vi "Get_FIFO.vi"(8 "error in (no error)":errorcluster) -> (0 "error out":errorcluster, 2 "TrajectoryFIFO":T1)   [LabVIEW 2019]
uses:
  <vilib>/Utility/error.llb/Error Cluster From Error Code.vi
  <vilib>/ErrorRing/Error Ring.xnode
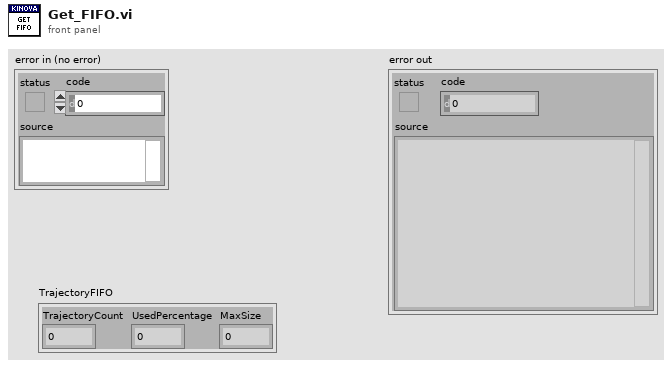
[diagram p1: front panel]
types:
  T1 = cluster{"TrajectoryCount":u32, "UsedPercentage":sgl, "MaxSize":u32}
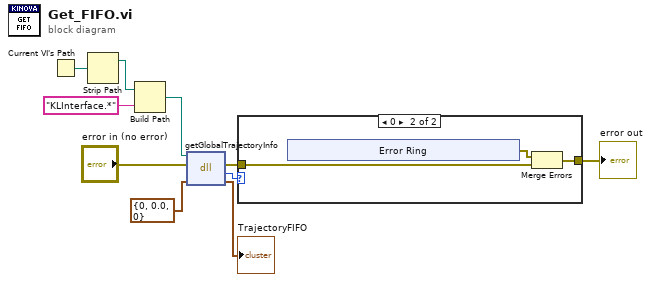
[diagram p0: block diagram]
diagram:
  n1 = Current VI's Path() -> (path=w7:path)
  n2 = Strip Path(path=w7) -> (stripped path=w6:path)  [unwired: 1 out]
  n3 = Build Path(base path=w6, name or relative path="KLInterface.*") -> (appended path=w2:path)
  n4 = dll-call lib="C:/Users/mcjssdcc/Documents/Kinova-Labview-Interface/KLInterface.dll" fn="getGlobalTrajectoryInfo"(path in=w2, error in="error in (no error)", "point"=T1 {"TrajectoryCount"=0, "UsedPercentage"=0.0, "MaxSize"=0} ("TrajectoryFIFO")) -> (error out=w9:errorcluster, "return type"=w8:i32, "point"=→"TrajectoryFIFO":T1)  [unwired: 1 in, 1 out]
  n5 = case shown="0" w8 {
    tunnel: [w11 w13] -> w5
    tunnel: w9 -> [w11 w12]
    frame 1, Default {
    }
    frame 0 {
      n6 = xnode "Error Ring"() -> ("error out"=w14:errorcluster)
      n7 = Merge Errors(w14, w12) -> (w13:errorcluster)
    }
  }
  "error out" <- w5
